vi "LVFunction_Imop_Compute_GaussianParameters.vi"(0 "HasoField in":refnum<class "HasoField.lvclass">, 5 "Path":path, 7 "nb_planes":i32, 9 "spottype":enum16{"square", "circle"}(ring), 11 "error in (no error)":errorcluster, 12 "degree":sgl) -> (4 "HasoField out":refnum<class "HasoField.lvclass">, 6 "Gaussian Param":T1, 15 "error out":errorcluster)   [LabVIEW 2018]
doc: "Gaussian parameters function.\n\n--------------------------------------------------------------------------------\n\n<B>config_file_pathIn</B> : Absolute path to the Haso configuration file.\n\n<B>config_file_pathOut</B> : Absolute path to the Haso configuration file.\n\n<B>HasoField</B> : HasoField object.\n\n<B>nb_planes</B> : Number of planes.\n\n<B>waist_position_millimeter</B> : Waist position (mm).\n\n<B>waist_radius_millimeter</B> : Waist radius (mm).\n\n<B>rayleigh_length_millimeter</B> : Rayleigh length (mm).\n\n<B>divergence</B> : Mivergence of the beam.\n\n<B>msquared</B> : m squared parameter.\n\n<B>spottype</B> : \"square\" or \"circle\" spot shape.\n\n<B>degree</B> : Angle of the square spot shape forms with an horizontal axis (degree).\n\n<B>ErrorIn</B> : Error\n\n<B>ErrorOut</B> : Error"
uses:
  Classes/HasoField/HasoField.lvclass
  Classes/HasoField/LVClass_HasoField Read HasoField.vi
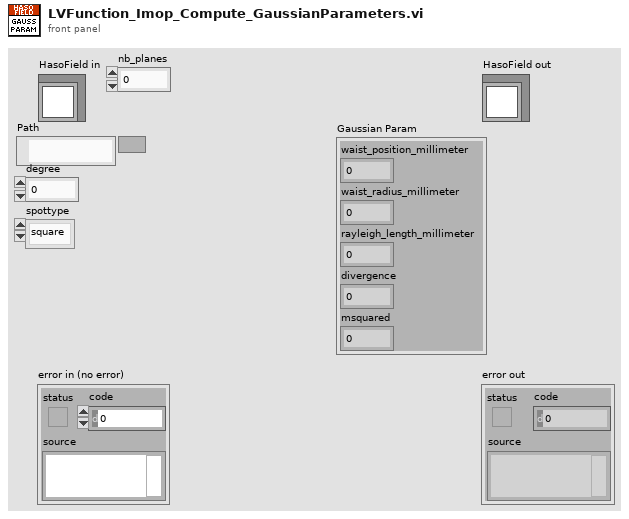
[diagram p1: front panel]
types:
  T1 = cluster{"waist_position_millimeter":sgl, "waist_radius_millimeter":sgl, "rayleigh_length_millimeter":sgl, "divergence":sgl, "msquared":sgl}
  T2 = typedef "ClassID.ctl" = i64
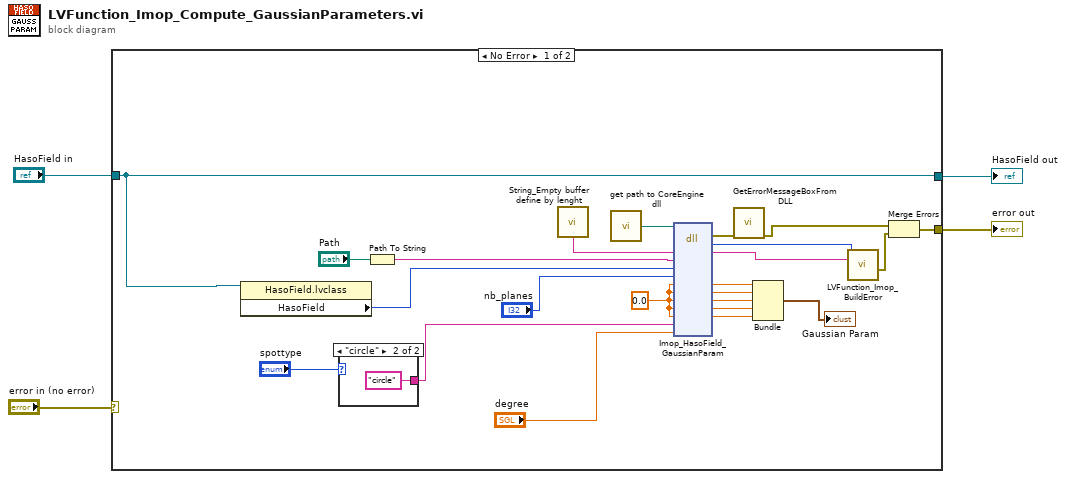
[diagram p0: block diagram]
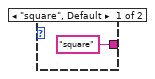
[diagram p2: hidden frame]
diagram:
  n1 = case shown="No Error" "error in (no error)" {
    selector: "error in (no error)" -> [_ w30]
    tunnel: "HasoField in" -> [w9 w31]
    tunnel: [w9 w31] -> w4
    tunnel: [w23 w30] -> w2
    frame No Error {
      w16 = sgl 0.0 ("waist_position_millimeter")
      n2 = property class="HasoField.lvclass"(reference=w9) -> ("HasoField"=w8:T2)  [unwired: 1 in, 2 out]
      n3 = case shown="\"circle\"" "spottype" {
        tunnel: ["square" "circle"] -> w5
        frame "square", Default {
        }
        frame "circle" {
        }
      }
      n4 = Path To String(path="Path") -> (string=w18:string)
      n5 = call "String_Empty buffer define by lenght.vi"() -> ("Empty buffer"=w22:string)  [unwired: 1 in]
      n6 = call "get path to CoreEngine dll.vi"() -> ("path to wavekit library"=w21:path)  [unwired: 14 in, 1 out]
      n7 = dll-call lib="D:/2_trunk/Soft_haso/ImOpCoreEngine4_LV2011/DLLs/ImopEngine4_vc100.dll" fn="Imop_HasoField_GaussianParam"(path in=w21, "message"=w22, "config file"=w18, "HasoField"=w8, "nb_planes"="nb_planes", "waist_position_millimeter"=w16, "waist_radius_millimeter"=w16, "rayleigh_length_millimeter"=w16, "divergence"=w16, "msquared"=w16, "spottype"=w5, "degree"="degree") -> (error out=w20:errorcluster, "return type"=w26:i32, "message"=w27:string, "waist_position_millimeter"=w15:sgl, "waist_radius_millimeter"=w14:sgl, "rayleigh_length_millimeter"=w13:sgl, "divergence"=w12:sgl, "msquared"=w11:sgl)  [unwired: 7 in, 1 out]
      n8 = call "GetErrorMessageBoxFromDLL.vi"("error IN"=w20) -> ("error OUT"=w25:errorcluster)  [unwired: 10 in]
      n9 = Bundle("waist_position_millimeter"=w15, "waist_radius_millimeter"=w14, "rayleigh_length_millimeter"=w13, "divergence"=w12, "msquared"=w11) -> (→"Gaussian Param":T1)  [unwired: 1 in]
      n10 = call "LVFunction_Imop_BuildError.vi"("code"=w26, "String to Prepend to source (\"\")"=w27) -> ("error out"=w24:errorcluster)  [unwired: 13 in]
      n11 = Merge Errors(w25, w24) -> (w23:errorcluster)
    }
    frame Error {
    }
  }
  "error out" <- w2
  "HasoField out" <- w4
